vi "Unpack Message.vi"(8 "error in (no error)":errorcluster, 9 "Packed Message":string, 10 "Message Name":string, 11 "Message Boolean in":refnum<class "Message Boolean.lvclass">) -> (0 "error out":errorcluster, 2 "Valid":bool, 3 "Message Boolean out":refnum<class "Message Boolean.lvclass">)   [LabVIEW 2016, in "Stream Mediator.lvlib" / "Message Boolean.lvclass"]
uses:
  <userlib>/Composed Systems/Stream/Mediator/Classes/Message Boolean/Message Boolean.lvclass
  C:/Program Files (x86)/National Instruments/LabVIEW 2016/user.lib/Composed Systems/Stream/Mediator/Classes/Message Interface/Message Interface.lvclass
  <userlib>/Composed Systems/Stream/Mediator/Classes/Message Boolean/Message Boolean.lvclass/Message Boolean.ctl
  <userlib>/Composed Systems/Stream/Mediator/Classes/Message Interface/Message Interface.lvclass
  <vilib>/addons/_JKI.lib/Serialization/JSON/JKI JSON Serialization.lvlib
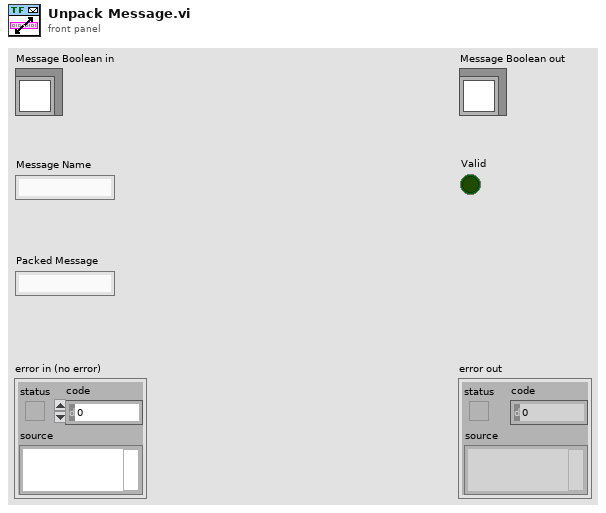
[diagram p1: front panel]
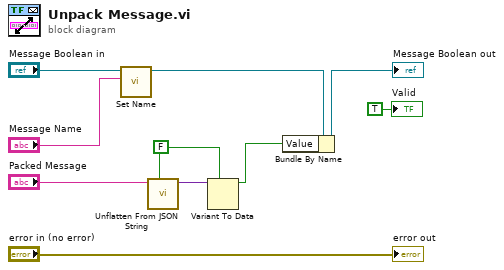
[diagram p0: block diagram]
diagram:
  w5 = FALSE
  n1 = call <userlib>:"Set Name.vi"("Name"="Message Name", "Message Interface in"="Message Boolean in") -> ("Message Interface out"=w8:refnum<class "Message Boolean.lvclass">)  [unwired: 8 in, 1 out]
  n2 = call <vilib>:"Unflatten From JSON String.vi"("Type and Defaults"=w5, "JSON String"="Packed Message") -> ("Variant"=w6:variant)  [unwired: 8 in, 1 out]
  n3 = Variant To Data(type=w5, Variant=w6) -> (data=w2:bool)  [unwired: 1 in, 1 out]
  n4 = Bundle By Name(cluster=w8, "Value"=w2) -> (→"Message Boolean out":refnum<class "Message Boolean.lvclass">)
  "error out" <- "error in (no error)"
  "Valid" <- TRUE ("Valid")
